vi "Run_Module.vi"(0 "VI_In":refnum<vi>, 11 "Error_In":errorcluster) -> (4 "VI_Out":refnum<vi>, 15 "Error_Out":errorcluster)   [LabVIEW 2023]
doc: "Used to run a VI From Another VI"
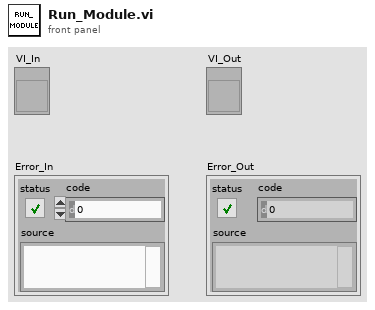
[diagram p1: front panel]
types:
  T1 = enum32{"Bad", "Idle", "Run top level", "Running"}
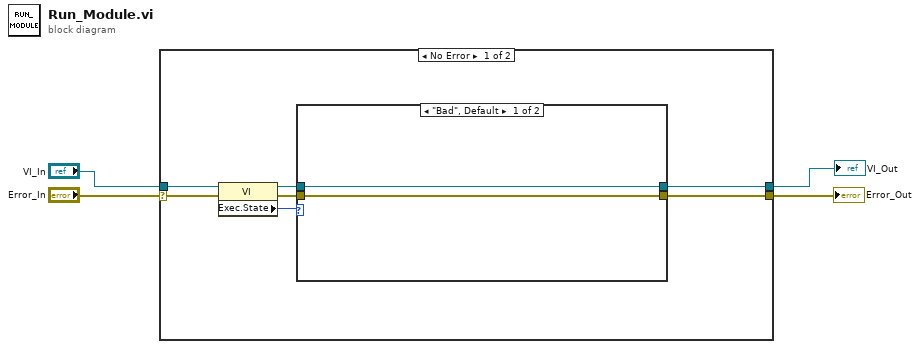
[diagram p0: block diagram]
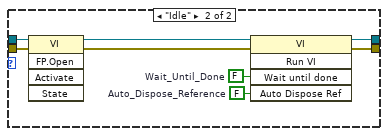
[diagram p2: hidden frame]
diagram:
  n1 = case shown="No Error" "Error_In" {
    selector: "Error_In" -> [w5 w23]
    tunnel: "VI_In" -> [w8 w22]
    tunnel: [w7 w22] -> w3
    tunnel: [w6 w23] -> w2
    frame No Error {
      n2 = property class="VI"(reference=w8, error in=w5) -> (reference out=w9:refnum<vi>, error out=w10:errorcluster, "Exec.State"=w11:T1)
      n3 = case shown="\"Bad\", Default" w11 {
        tunnel: [w13 w17] -> w6
        tunnel: [w12 w16] -> w7
        tunnel: w9 -> [w12 w15]
        tunnel: w10 -> [w13 w14]
        frame "Bad", Default {
        }
        frame "Idle" {
          w21 = FALSE  # Auto_Dispose_Reference
          w20 = FALSE  # Wait_Until_Done
          n4 = invoke on="Invoke Node" class="VI" method="FP.Open"(reference=w15, error in=w14) -> (reference out=w19:refnum<vi>, error out=w18:errorcluster)  [unwired: 3 in, 3 out]
          n5 = invoke on="Invoke Node" class="VI" method="Run VI"(reference=w19, error in=w18, "Wait until done"=w20, "Auto Dispose Ref"=w21) -> (reference out=w16:refnum<vi>, error out=w17:errorcluster)  [unwired: 1 in, 3 out]
        }
      }
    }
    frame Error {
    }
  }
  "VI_Out" <- w3
  "Error_Out" <- w2
